vi "Write Display Control.vi"(8 "error in (no error)":errorcluster, 9 "Display Control":T1, 10 "VISA resource name in":refnum<visa-resource-name>, 11 "LCD-I2C in":refnum<class "LCD-I2C.lvclass">) -> (0 "error out":errorcluster, 2 "VISA resource name":refnum<visa-resource-name>, 3 "LCD-I2C out":refnum<class "LCD-I2C.lvclass">)   [LabVIEW 2023, in "CTI-Visa-DeviceLib.lvlib" / "LCD-I2C.lvclass"]
uses:
  LCD-I2C.lvclass
  Display Control.ctl
  Command.ctl
  LCD-I2C.lvclass/LCD-I2C.ctl
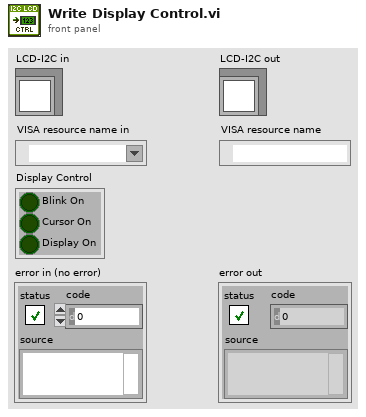
[diagram p1: front panel]
types:
  T1 = typedef "CTI-Visa-DeviceLib.lvlib/LCD-I2C.lvclass/Display Control.ctl" = cluster{"Blink On":bool, "Cursor On":bool, "Display On":bool}
  T2 = typedef "CTI-Visa-DeviceLib.lvlib/LCD-I2C.lvclass/Command.ctl" = enum16{"Clear Display", "Return Home", "Entry Mode Set", "Display Control", "Cursor Shift", "Function Set", "Set CGRAM Addr", "Set DDRAM Addr"}
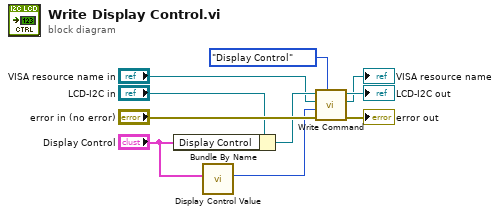
[diagram p0: block diagram]
diagram:
  n1 = Bundle By Name(cluster="LCD-I2C in", "Display Control"="Display Control") -> (w7:refnum<class "LCD-I2C.lvclass">)
  n2 = call "Display Control Value.vi"("Display Control"="Display Control") -> ("DCtrl Value"=w1:u8)  [unwired: 10 in]
  n3 = call "Write Command.vi"("Command"=Command."Display Control", "error in (no error)"="error in (no error)", "Value"=w1, "VISA resource name in"="VISA resource name in", "LCD-I2C in"=w7) -> ("error out"=→"error out":errorcluster, "VISA resource name"=→"VISA resource name":refnum<visa-resource-name>, "LCD-I2C out"=→"LCD-I2C out":refnum<class "LCD-I2C.lvclass">)  [unwired: 4 in]
